vi "FLAGSdll.vi"(8 "error in (no error)":errorcluster, 10 "jFlag":i32=-999, 11 "hFlag":string) -> (0 "error out":errorcluster, 3 "Outputs":T1)   [LabVIEW 2015]
doc: "subroutine FLAGSdll(hFlag, jFlag, kFlag, ierr, herr, hFlag_length, herr_length)\n\nSet flags for desired behavior from the program.\n\nINPUTS:\nhFlag -- Indicator for the option to set (letters in the string are case insensitive).\njFlag -- Flag to choose what to do in each option. Send -999 to just obtain the current value of the flag.\n\nOUTPUTS:\nkFlag -- Current setting of the flag for the option identified by iFlag. (Returned regardless of the value of jFlag.)\nierr -- Error flag\nherr -- Error string (character*255)\nhFlag_length -- length of variable hFlag (default: 255)\nherr_length -- length of variable herr (default: 255)\n\nTable of flags in FLAGS function:\n\nhFlag jFlag\n________________________________________________________________________________________________________________\nReturn errors • 0 - Return only final messages (default).\nor Errors • 1 - Return all intermediate messages.\n • 2 - Do not return messages.\n This flag is not reset with a new call to SETUP.\n\nWrite errors • 0 - Error strings not written to screen (default).\nor Write • -1 - Error string written to screen.\n • 1 - Error string written to screen only if ierr is positive.\n • 3,-3 - Same as 1 and -1, but program also pauses.\n This flag is not reset with a new call to SETUP.\n\nDir search • 0 - Search for fluid files in alternate directories (as defined in \nor Dir OPENFL) (default).\n • 1 - Do not search in directories other than the one set by the \n call to SETPATH, except for a ‘fluids’ subdirectory within the \n folder given in SETPATH. If the fluid files for the reference \n fluid(s) are not in the SETPATH directory, then transport \n properties may not be calculated.\n • 2 - Make no additional checks if the fluid file is not found \n after the first attempt to open the file (for example, checking \n upper and lower case). This flag is never reset.\n\nSkip SETREF • 0 - Call the SETREF routine to setup the reference state \nor Skip (default).\n • 1 - Skip the call to SETREF. However, this means energy, \n enthalpy, and entropy will not be correct (but only by an offset \n to their usual values). This must be called before the call to \n SETUP, and is never reset.\n\nMixture reference • 0 - Do nothing (default).\nor SETREF • 2 - When calling subroutine REFPROP, call SETREF first with a \n value of 2 for the second entry. (See subroutine SETREF for \n details.) This must be called before the call to REFPROP (the \n subroutine in PROP_SUB.FOR), and is never reset.\n\nSkip ECS • 0 - Load the ECS fluids required for transport properties (for \n pure fluids in slots 21-40 and mixtures in slot 41).\n • 1 - Don’t load the ECS fluids, only the requested fluids (this \n may deactivate pure fluid transport properties, and will \n deactivate all mixture transport calculations. This must be \n called before the call to SETUP, and is never reset. Splines off \n • 1 - Turn the splines off (assuming that they were turned on \n initially by a call to SATSPLN). Calling SETUP again will also \n turn off the splines.\n\nIgnore bounds • 0 - Check all errors and respond accordingly (default).\nor Bounds • 1 - Ignore bounds for certain situations, such as calling SATT \n below the triple point or states above the melting line. This \n flag is never reset.\n\nCache • 0 - Cache all calculated values (default).\n • 1 - Cache only low level calculations, such as derivatives \n calculated in PHIFEQ.\n • 2 - Cache only calculated properties in major subroutines \n such as SATT and SATP.\n • 3 - No caching. This flag is not reset with a new call to SETUP.\n\nReset all • 2 - Call RESETA to reset all cached values. This includes all \n flags set by calls to this or RA routine, except for the use of a \n pure fluid in a mixture or reducing nc. Subroutine RESETA is \n always called by SETUP, but does not reset the flags set by \n calls to this routine.\n\nPure fluid • 0 - Use full mixture equation of state loaded (default).\nor Pure • <>0 - Use the pure fluid loaded in the slot specified by jFlag. \n This option is reset during the call to SETUP. Component \n number or nc. \n • nc - Reduce the number of fluids being used to nc. See SETNC \n routine for details. The output in kFlag will give the number of \n fluids in use, which can be useful even if this option has not \n been called to set nc.This option is reset during the call to \n SETUP.\n\nPeng-Robinson • 0 - Turn off the Peng-Robinson equation of state (default).\nor PR • 2 - Use Peng-Robinson equation for all calculations.\n • 3 - Use Peng-Robinson with translation term deactivated. This \n option is reset during the call to SETUP.\n\nkij Zero • 0 - Use the fitted kij values found in the HMX.BNC file on the \n lines with PR1 (default).\n • 1 - Set all kij values to those estimated in ESTPR (thus ignoring \n the ones on the PR1 lines in the HMX.BNC file).\n • 2 - Set all kij values to zero. This option is never reset.\n\nAGA8 • 0 - Turn off AGA8 and return to the fluids loaded from the call \n to SETUP (default)\n • 1 - Turn on the use of the AGA8 DETAIL equation of state. This \n option is reset during the call to SETUP.\n\nGERG 2008 • 0 - Set a flag to turn off GERG 2008 next time SETUP is called.\nor GERG • 1 - Turn on the flag that will cause the GERG 2008 equation to \n be loaded next time SETUP is called This option MUST be \n called before SETUP. When turning off the GERG, call the \n SETUP routine again after calling this routine.\n\nGas constant • 0 - Default is to use the most current gas constant for all \n fluids except nitrogen, argon,or R oxygen, ethylene, CO2, \n methane, and ethane.\n • 1 - Use most current gas constant for all fluids (must be \n called after call to SETUP).\n • 2 - Use gas constant from fluid files for each equation of state \n (must be called after call to SETUP). This option is reset during \n the call to SETUP.\n\nCalorie • 0 - Use a calorie to joule conversion value of 4.184 cal/J \nor Cal (default).\n • 1 - Use the IT value of 4.1868 cal/J. This option is never reset.\n\nDebug • 0 - Turn off all debugging.\n • 1 - In the REFPROP subroutine, write all input variables to a \n file called input.dat, and all output values to a file called \n output.dat\n • 2 - In SETUP, write out the full path of the files that were \n either opened or tried to open. This option is never reset."
uses:
  REFPROP.dll
panel:
  # "REFPROP-FLAGSdll.vi"
  # "void  FLAGSdll(CStr hFlag, CStr jFlag, int32_t *ierr, CStr herr, int32_t herr length);"
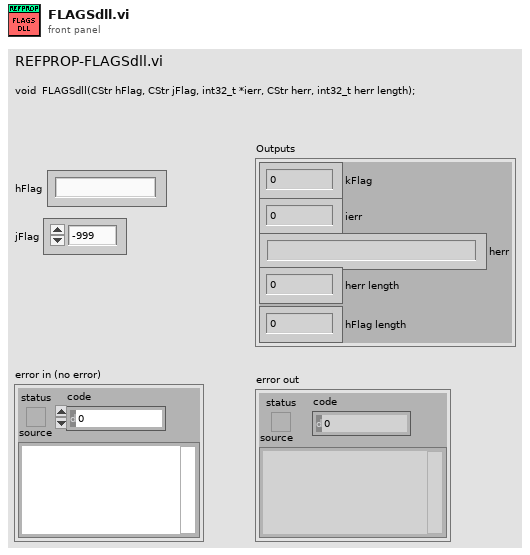
[diagram p1: front panel]
types:
  T1 = cluster{"kFlag":i32, "ierr":i32, "herr":string, "herr length":i32, "hFlag length":i32}
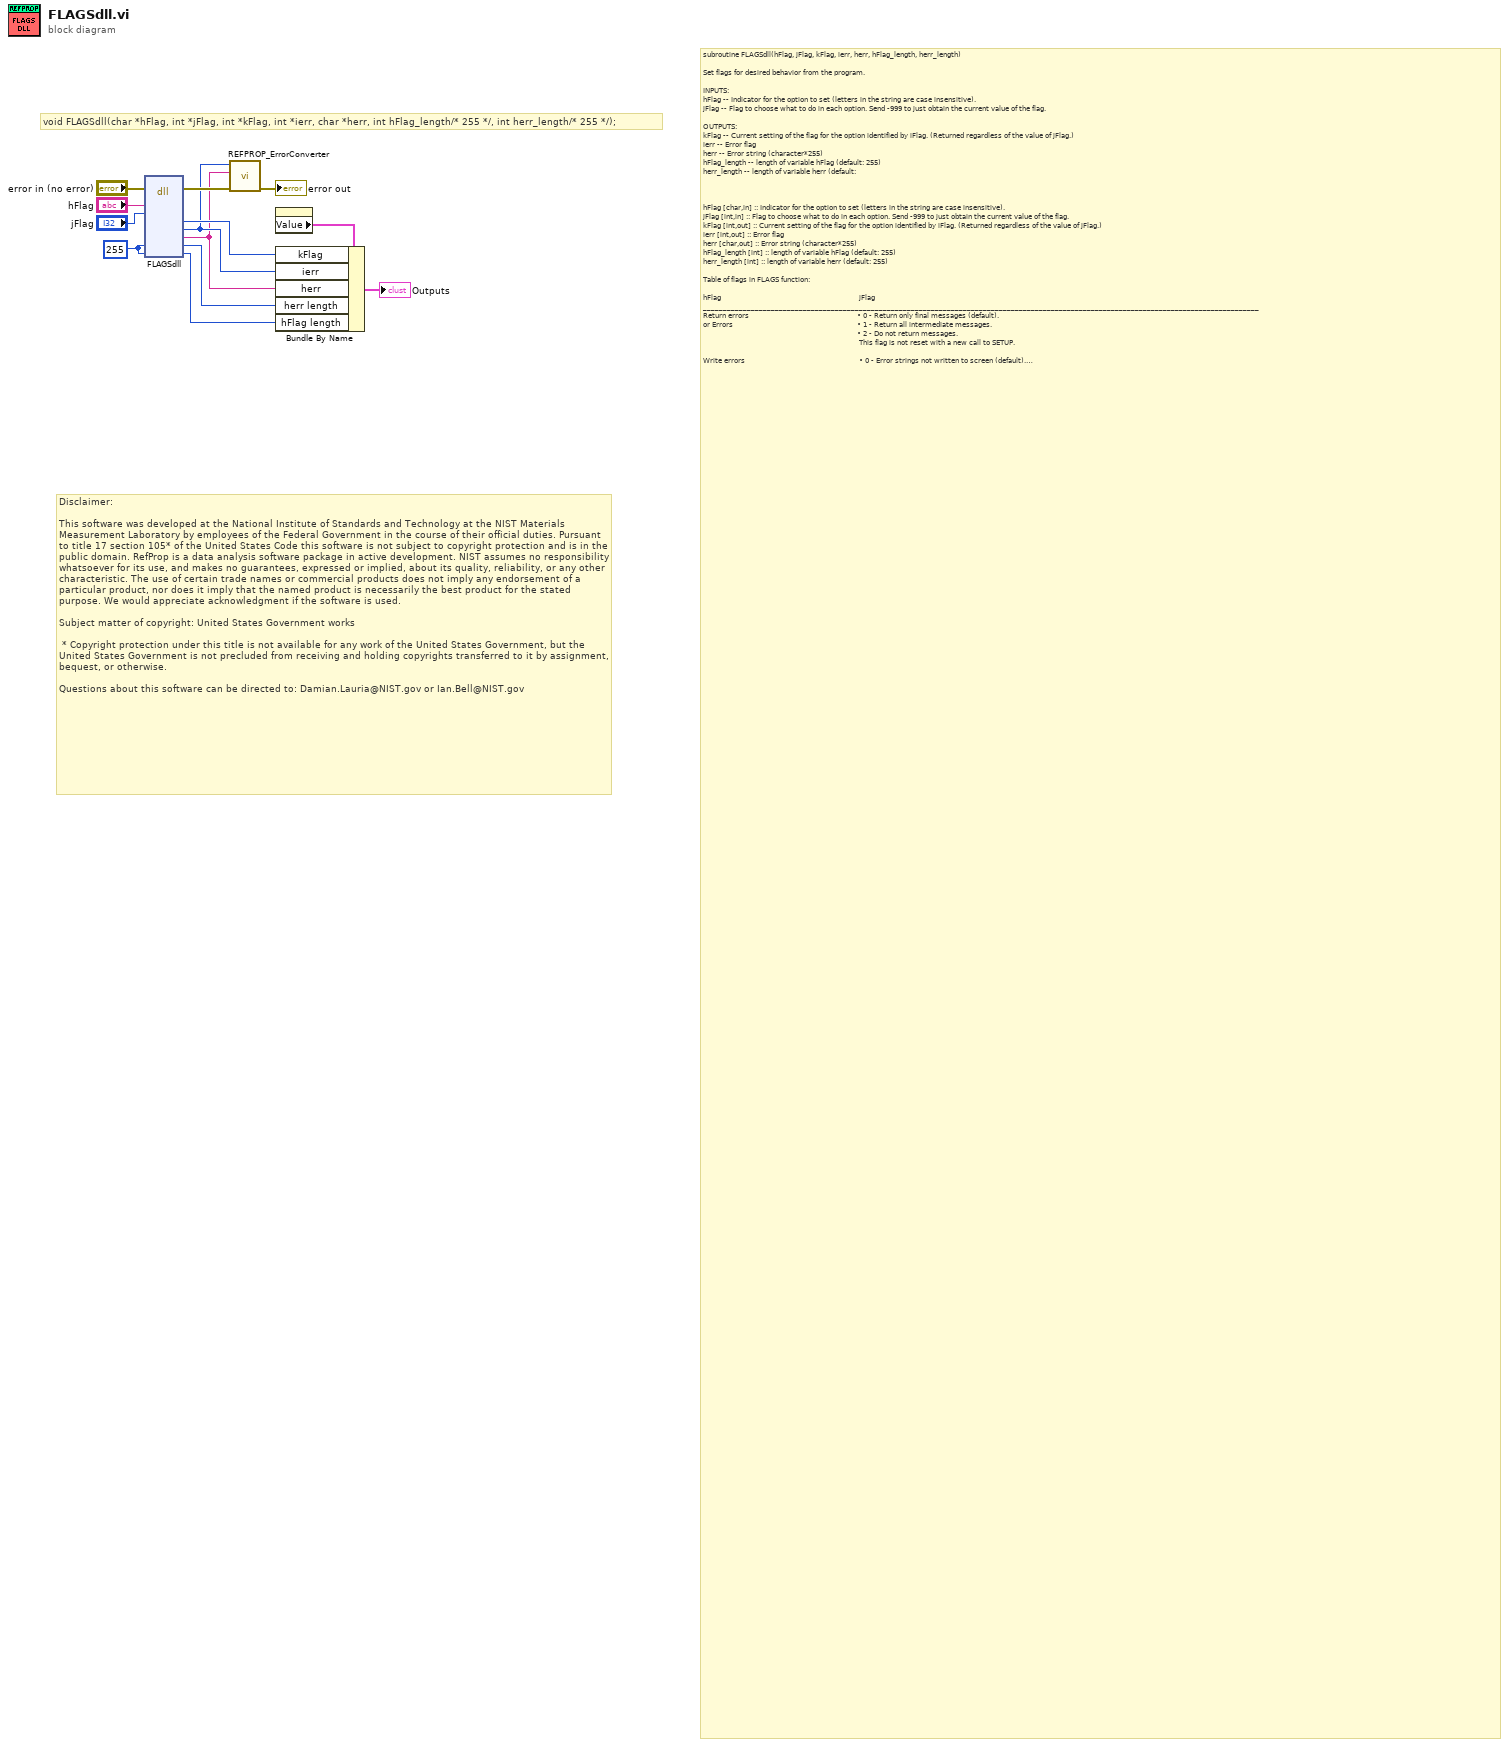
[diagram p0: block diagram]
diagram:
  w8 = 255 ("hFlag length")
  # "void FLAGSdll(char *hFlag, int *jFlag, int *kFlag, int *ierr, char *herr, int hFlag_length/* 255 */, int herr_length/* 255 */);"
  # "Disclaimer:\n\nThis software was developed at the National Institute of Standards and Technology at the NIST Materials Measurement Laboratory by employees of the Federal Government in the course of their official duties. Pursuant to title 17 section 105* of the United States Code this software is not subject to copyright protection and is in the public domain. RefProp is a data analysis software package in active development. NIST assumes no responsibility whatsoever for its use, and makes no guarantees, expressed or implied, about its quality, reliability, or any other characteristic. The use of certain trade names or commercial products does not imply any endorsement of a particular product, nor does it imply that the named product is necessarily the best product for the stated purpose. We would appreciate acknowledgment if the software is used.\n \nSubject matter of copyright: United States Government works\n  \n * Copyright protection under this title is not available for any work of the United States Government, but the United States Government is not precluded from receiving and holding copyrights transferred to it by assignment, bequest, or otherwise.\n\nQuestions about this software can be directed to: Damian.Lauria@NIST.gov or Ian.Bell@NIST.gov"
  # "subroutine FLAGSdll(hFlag, jFlag, kFlag, ierr, herr, hFlag_length, herr_length)\n\nSet flags for desired behavior from the program.\n\nINPUTS:\nhFlag -- Indicator for the option to set (letters in the string are case insensitive).\njFlag -- Flag to choose what to do in each option. Send -999 to just obtain the current value of the flag.\n\nOUTPUTS:\nkFlag -- Current setting of the flag for the option identified by iFlag. (Returned regardless of the value of jFlag.)\nierr -- Error flag\nherr -- Error string (character*255)\nhFlag_length -- length of variable hFlag (default: 255)\nherr_length -- length of variable herr (default: \n\n\n\nhFlag [char,in] :: Indicator for the option to set (letters in the string are case insensitive).\njFlag [int,in] :: Flag to choose what to do in each option. Send -999 to just obtain the current value of the flag.\nkFlag [int,out] :: Current setting of the flag for the option identified by iFlag. (Returned regardless of the value of jFlag.)\nierr [int,out] :: Error flag\nherr [char,out] :: Error string (character*255)\nhFlag_length [int] :: length of variable hFlag (default: 255)\nherr_length [int] :: length of variable herr (default: 255)\n\nTable of flags in FLAGS function:\n\nhFlag                                                                     jFlag\n___________________________________________________________________________________________________________________________________________\nReturn errors                                                      • 0 - Return only final messages (default).\nor Errors                                                              • 1 - Return all intermediate messages.\n                                                                             • 2 - Do not return messages.\n                                                                              This flag is not reset with a new call to SETUP.\n\nWrite errors                                                         • 0 - Error strings not written to screen (default).\nor Write                                                               • -1 - Error string written to screen.\n                                                                             • 1 - Error string written to screen only if ierr is positive.\n                                                                             • 3,-3 - Same as 1 and -1, but program also pauses.\n                                                                                This flag is not reset with a new call to SETUP.\n\nDir search                                                            • 0 - Search for fluid files in alternate directories (as defined in OPENFL) (default).\nor Dir                                                                    • 1 - Do not search in directories other than the one set by the call to SETPATH, except\n                                                                                for a ‘fluids’ subdirectory within the folder given in SETPATH. If the fluid files for the\n                                                                                reference fluid(s) are not in the SETPATH directory, then transport properties may not \n                                                                                be calculated.\n                                                                             • 2 - Make no additional checks if the fluid file is not found after the first attempt to                      \n                                                                                open the file (for example, checking upper and lower case). This flag is never reset.\n\nSkip SETREF                                                        • 0 - Call the SETREF routine to setup the reference state (default).\nor Skip                                                                 • 1 - Skip the call to SETREF. However, this means energy, enthalpy, and entropy will not \n                                                                                be correct (but only by an offset to their usual values). This must be called before the \n                                                                                call to SETUP, and is never reset.\n\nMixture reference                                              • 0 - Do nothing (default).\nor SETREF                                                           • 2 - When calling subroutine REFPROP, call SETREF first with a value of 2 for the second \n                                                                                entry. (See subroutine SETREF for details.) This must be called before the call to \n                                                                                REFPROP (the subroutine in PROP_SUB.FOR), and is never reset.\n\nSkip ECS                                                             • 0 - Load the ECS fluids required for transport properties (for pure fluids in slots 21-40 \n                                                                              and mixtures in slot 41).\n                                                                            • 1 - Don’t load the ECS fluids, only the requested fluids (this may deactivate pure fluid  \n                                                                               transport properties, and will deactivate all mixture transport calculations. This must be \n                                                                               called before the call to SETUP, and is never reset. \n\nSplines off                                                          • 1 - Turn the splines off (assuming that they were turned on initially by a call to \n                                                                               SATSPLN). Calling SETUP again will also turn off the splines.\n\nIgnore bounds                                                  • 0 - Check all errors and respond accordingly  (default).\nor Bounds                                                          • 1 - Ignore bounds for certain situations, such as calling SATT below the triple point or \n                                                                               states above the melting line. This flag is never reset.\n\nCache                                                                 • 0 - Cache all calculated values (default).\n                                                                            • 1 - Cache only low level calculations, such as derivatives calculated in PHIFEQ.\n                                                                            • 2 - Cache only calculated properties in major subroutines such as SATT and SATP.\n                                                                            • 3 - No caching. This flag is not reset with a new call to SETUP.\n\nReset all                                                              • 2 - Call RESETA to reset all cached values. This includes all flags set by calls to this \nor RA                                                                    routine, except for  the use of a pure fluid in a mixture or reducing nc. Subroutine  \n                                                                              RESETA is always called by SETUP, but does not reset the flags set by calls to this \n                                                                              routine.\n\nPure fluid                                                           • 0 - Use full mixture equation of state loaded (default).\nor Pure                                                               • <>0 - Use the pure fluid loaded in the slot specified by jFlag. This option is reset  \n                                                                                during the call to SETUP. Component number or nc \n                                                                            • nc - Reduce the number of fluids being used to nc. See SETNC routine for details. The \n                                                                              output in kFlag will give the number of fluids in use, which can be useful even if this  \n                                                                              option has not been called to set nc.This option is reset during the call to SETUP.\n\nPeng-Robinson                                                 • 0 - Turn off the Peng-Robinson equation of state (default).\nor PR                                                                   • 2 - Use Peng-Robinson equation for all calculations.\n                                                                            • 3 - Use Peng-Robinson with translation term deactivated. This option is reset during the \n                                                                               call to SETUP.\n\nkij Zero                                                               • 0 - Use the fitted kij values found in the HMX.BNC file on the lines with PR1 (default).\n                                                                            • 1 - Set all kij values to those estimated in ESTPR (thus ignoring the ones on the PR1 lines \n                                                                              in the HMX.BNC file).\n                                                                            • 2 - Set all kij values to zero. This option is never reset.\n\nAGA8                                                                  • 0 - Turn off AGA8 and return to the fluids loaded from the call to SETUP (default)\n                                                                            • 1 - Turn on the use of the AGA8 DETAIL equation of state. This option is reset during \n                                                                               the call to SETUP.\n\nGERG 2008                                                          • 0 - Set a flag to turn off GERG 2008 next time SETUP is called.\nor GERG                                                              • 1 - Turn on the flag that will cause the GERG 2008 equation to be loaded next time \n                                                                              SETUP is called This option MUST be called before SETUP. When turning off the GERG, \n                                                                              call the SETUP routine again after calling this routine.\n\nGas constant                                                      • 0 - Default is to use the most current gas constant for all fluids except nitrogen, argon,or R                                                                      \n                                                                               oxygen, ethylene, CO2, methane, and ethane.\n                                                                             • 1 - Use most current gas constant for all fluids (must be called after call to SETUP).\n                                                                             • 2 - Use gas constant from fluid files for each equation of state (must be called after call \n                                                                               to SETUP). This option is reset during the call to SETUP.\n\nCalorie                                                                 • 0 - Use a calorie to joule conversion value of 4.184 cal/J (default).\nor Cal                                                                   • 1 - Use the IT value of 4.1868 cal/J. This option is never reset.\n\nDebug                                                                  • 0 - Turn off all debugging.\n                                                                              • 1 - In the REFPROP subroutine, write all input variables to a file called input.dat, and all \n                                                                               output values to a file called output.dat\n                                                                              • 2 - In SETUP, write out the full path of the files that were either opened or tried to \n                                                                               open. This option is never reset."
  n1 = dll-call lib="C:/Users/lauria/Desktop/REFPROP 10 LabVIEW Wrapper BETA/REFPROP/REFPROP.*" fn="FLAGSdll"(error in="error in (no error)", "hFlag"="hFlag", "jFlag"="jFlag", "hFlag length"=w8, "herr length"=w8) -> (error out=w13:errorcluster, "kFlag"=w5:i32, "ierr"=w4:i32, "herr"=w3:string, "hFlag length"=w2:i32, "herr length"=w1:i32)  [unwired: 8 in, 1 out]
  n2 = call "REFPROP_ErrorConverter.vi"("error in (no error)"=w13, "Error Message"=w3, "Error Code"=w4) -> ("error out"=→"error out":errorcluster)  [unwired: 8 in]
  n3 = property on="Outputs" class="Clust (strict)"() -> ("Value"=w7:T1)  [unwired: 2 in, 2 out]
  n4 = Bundle By Name(cluster=w7, "kFlag"=w5, "ierr"=w4, "herr"=w3, "herr length"=w2, "hFlag length"=w1) -> (→"Outputs":T1)
